vi "Launch Nested Actors.vi"(8 "error in (no error)":errorcluster, 11 "Syringe in":refnum<class "Syringe Line.lvclass">) -> (0 "error out":errorcluster, 3 "Syringe out":refnum<class "Syringe Line.lvclass">)   [LabVIEW 2015, in "cRIO-Carbondioxide.lvlib" / "CO2-Actor.lvlib" / "Syringe Line.lvclass"]
uses:
  Syringe Line.lvclass
  <vilib>/ActorFramework/Actor/Actor.lvclass
  Valve/Action.ctl
  Valve/Valve.lvclass/Valve.ctl
  Syringe Line.lvclass/Syringe Line.ctl
  CO2 Actor/CO2 Actor.lvclass
  Valve/Valve.lvclass
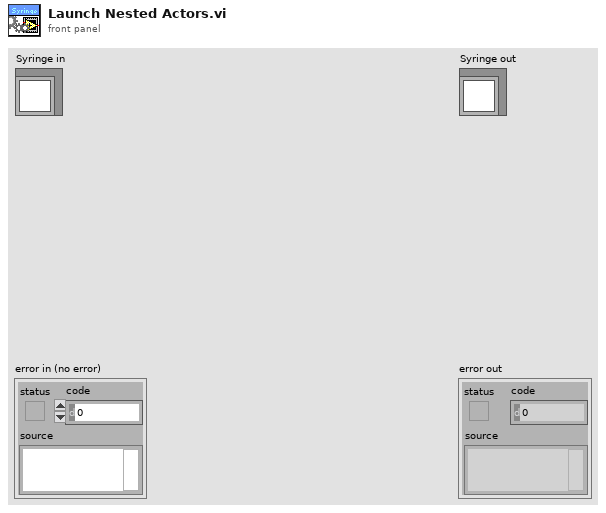
[diagram p1: front panel]
types:
  T1 = typedef "Action.ctl" = enum16{"Open", "Close", "None"}
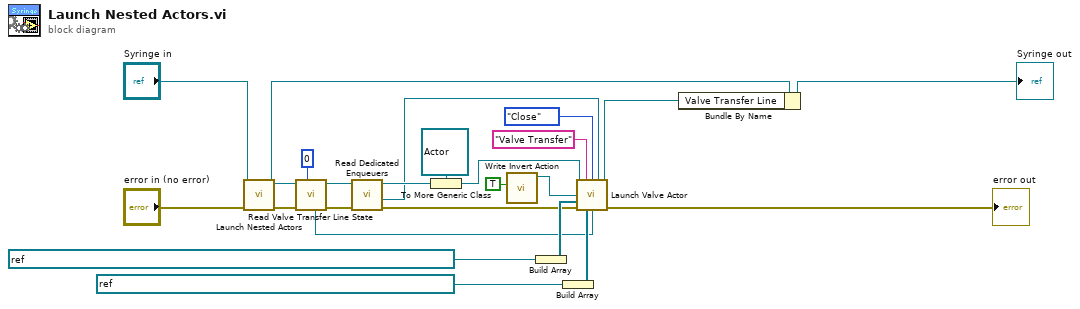
[diagram p0: block diagram]
diagram:
  n1 = call-parent "Launch Nested Actors.vi"("error in (no error)"="error in (no error)", "CO2 Actor in"="Syringe in") -> ("error out"=w7:errorcluster, "CO2 Actor out"=w9:refnum<class "Syringe Line.lvclass">)  [unwired: 8 in]
  n2 = call "Read Valve Transfer Line State.vi"("timeout in ms (-1)"=0, "error in (no error)"=w7, "Syringe Line in"=w9) -> ("error out"=w6:errorcluster, "Syringe Line out"=w8:refnum<class "Syringe Line.lvclass">, "Valve Syringe Line StateQ"=w5:refnum<queue>)  [unwired: 5 in, 1 out]
  n3 = call "Read Dedicated Enqueuers.vi"("error in (no error)"=w6, "CO2 Actor in"=w8) -> ("error out"=w11:errorcluster, "DedicatedEnQrs"=w10:refnum<queue>, "CO2 Actor out"=w12:refnum<class "Syringe Line.lvclass">)  [unwired: 6 in, 1 out]
  n4 = To More Generic Class(target class=refnum<class "Actor.lvclass"> refnum ("Caller Actor in"), reference=w12) -> (generic class reference=w3:refnum<class "Actor.lvclass">)
  n5 = call "Write Invert Action.vi"("Invert Action"=TRUE) -> ("Valve out"=w2:refnum<class "Valve.lvclass">)  [unwired: 10 in]
  n6 = Build Array(refnum<k21> "ni.var.psp://crio-carbondioxide/AMS Gas SHV/Valves/Syringe-Line Valve HV314" ("SHV")) -> (w13:refnum<k21>[])
  n7 = Build Array(refnum<k21> "ni.var.io://crio-carbondioxide/Mod1/Syringe-Line Valve HV314" ("SHV")) -> (w21:refnum<k21>[])
  n8 = call "Launch Valve Actor.vi"("Caller Actor in"=w3, "Name"="Valve Transfer", "Start Action (Open)"=Action."Close", "DedicatedEnQrs"=w10, "Valve in"=w2, "SHV Aliases"=w13, "error in (no error)"=w11, "SHV"=w21, "StateQ"=w5) -> ("Caller-To-Actor Enqueuer"=w15:refnum<class "Message Enqueuer.lvclass">, "error out"=→"error out":errorcluster)  [unwired: 5 in]
  n9 = Bundle By Name(cluster=w9, "Valve Transfer Line"=w15) -> (→"Syringe out":refnum<class "Syringe Line.lvclass">)
